vi "ActionVIOnCompile.vi"(8 "error in (no error)":errorcluster, 11 "Device Item Ref in":T1 format="%.0x") -> (0 "error out":errorcluster)   [LabVIEW 2027, in "System Monitor System Explorer.lvlib"]
uses:
  System Monitor System Explorer.lvlib
  <vilib>/NI VeriStand/Custom Device API/Custom Device Item Ref.ctl
  Shared/Compiled.Settings.ctl
  Shared/System Monitor Settings.ctl
  <vilib>/NI VeriStand/Custom Device API/Custom Device Loop Flags.ctl
  Shared/Constants.vi
  <vilib>/NI VeriStand/Custom Device API/Set Item Property (Variant).vi
  <vilib>/NI VeriStand/Custom Device API/Custom Device API.lvlib
  <vilib>/NI/NIVS Inline Async API/_Data Access System Explorer/Data Access System Explorer.lvlib
  Shared/System Monitor Shared.lvlib
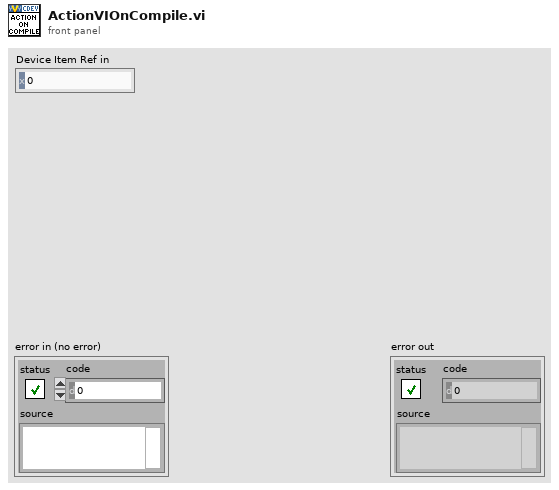
[diagram p1: front panel]
types:
  T1 = typedef "Custom Device API.lvlib/Custom Device Item Ref.ctl" = u64
  T2 = typedef "Custom Device API.lvlib/Custom Device Loop Flags.ctl" = cluster{"Disable \"Execute Model\"":bool, "Disable \"Read Data from HW\"":bool, "Disable \"Write Data to HW\"":bool}
  T3 = typedef "System Monitor Shared.lvlib/Compiled.Settings.ctl" = cluster{"Name":string, "System Monitor Settings":T4}
  T4 = typedef "System Monitor Shared.lvlib/System Monitor Settings.ctl" = cluster{"Number of CPU Cores":u64, "Update Rate (Hz)":dbl}
  T5 = enum16{"Output/Write", "Input/Read", "Input/ReadWrite"}
  T6 = cluster{"Name":string, "Type":enum16{"Output/Write", "Input/Read", "Input/ReadWrite"}, "VS Refs":T1[]}
  T7 = typedef "Custom Device API.lvlib/Custom Device Item Info.ctl" = cluster{"Name":string, "Is Channel":bool, "GUID":string, "Is Waveform":bool}
  T8 = cluster{"Name":string, "Type":enum16{"Output/Write", "Input/Read", "Input/ReadWrite"}, "VS Refs":T1[]}[]
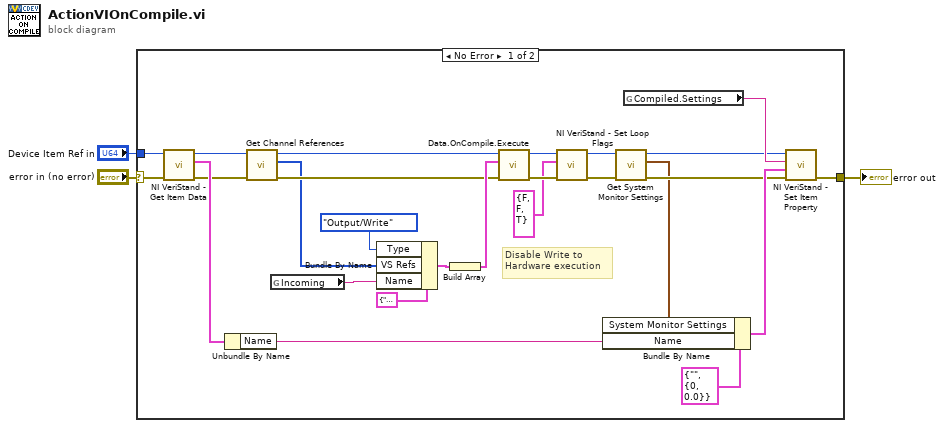
[diagram p0: block diagram]
diagram:
  n1 = case shown="No Error" "error in (no error)" {
    selector: "error in (no error)" -> [w27 w30]
    tunnel: [w28 w30] -> w2
    tunnel: "Device Item Ref in" -> [w26 _]
    frame No Error {
      # "Disable Write to\nHardware execution"
      n2 = call <vilib>:"NI VeriStand - Get Item Data.vi"("error in (no error)"=w27, "Item Ref in"=w26) -> ("error out"=w12:errorcluster, "Item Info"=w25:T7, "Item Ref out"=w13:T1)  [unwired: 6 in, 1 out]
      n3 = Unbundle By Name(w25) -> ("Name"=w24:string)
      n4 = call "Get Channel References.vi"("error in (no error)"=w12, "Item Ref in"=w13) -> ("error out"=w10:errorcluster, "Channel Refs out"=w8:T1[], "Item Ref out"=w11:T1)  [unwired: 7 in]
      n5 = global read "Constants.vi" "Incoming"() -> (w9:string)
      n6 = Bundle By Name(cluster=T6 {"Name"="", "Type"=enum."Output/Write", "VS Refs"=[]} ("Group"), "Type"=T5."Output/Write", "VS Refs"=w8, "Name"=w9) -> (w20:T6)
      n7 = Build Array(w20) -> (w22:T8)
      n8 = call <vilib>:"Data.OnCompile.Execute.vi"("error in"=w10, "VS Ref Groups"=w22, "Custom Device Ref"=w11) -> ("error out"=w6:errorcluster, "Custom Device Ref"=w19:T1)  [unwired: 7 in]
      n9 = call <vilib>:"NI VeriStand - Set Loop Flags.vi"("error in (no error)"=w6, "Loop Flags"=T2 {"Disable \"Execute Model\""=FALSE, "Disable \"Read Data from HW\""=FALSE, "Disable \"Write Data to HW\""=TRUE}, "Item Ref in"=w19) -> ("error out"=w5:errorcluster, "Item Ref out"=w7:T1)  [unwired: 7 in]
      n10 = call "Get System Monitor Settings.vi"("error in (no error)"=w5, "Item Ref in"=w7) -> ("error out"=w15:errorcluster, "System Monitor Settings"=w14:T4, "Item Ref out"=w16:T1)  [unwired: 7 in]
      n11 = Bundle By Name(cluster=T3 {"Name"="", "System Monitor Settings"={"Number of CPU Cores"=0, "Update Rate (Hz)"=0.0}} ("Compiled.Settings"), "System Monitor Settings"=w14, "Name"=w24) -> (w29:T3)
      n12 = global read "Constants.vi" "Compiled.Settings"() -> (w17:string)
      n13 = call-poly <vilib>:"NI VeriStand - Set Item Property.vi"("error in (no error)"=w15, "Value"=w29, "Property Name"=w17, "Item Ref in"=w16) -> ("error out"=w28:errorcluster)  [unwired: 5 in, 2 out]
    }
    frame Error {
    }
  }
  "error out" <- w2
